vi "Base Ctrl Start Values.vi"(0 "Notifier Name In":string, 11 "Error In":errorcluster) -> (2 "Turret Filter":u32, 3 "Obj Index":u32, 4 "Notifier Name Out":string, 6 "Output Port":u32, 8 "Lamp Power":dbl, 10 "Lamp State":bool, 15 "Error Out":errorcluster)   [LabVIEW 2020]
uses:
  Device Library/Microscopes/Polymorphic Microscope Messenger/Get Turret Filter.vi
  Device Library/Microscopes/Polymorphic Microscope Messenger/Get Obj Index.vi
  Device Library/Microscopes/Polymorphic Microscope Messenger/Set Lamp Index.vi
  Device Library/Microscopes/Polymorphic Microscope Messenger/Get Output Port.vi
  Device Library/Microscopes/Polymorphic Microscope Messenger/Get Lamp Power.vi
  Device Library/Microscopes/Polymorphic Microscope Messenger/Get Lamp State.vi
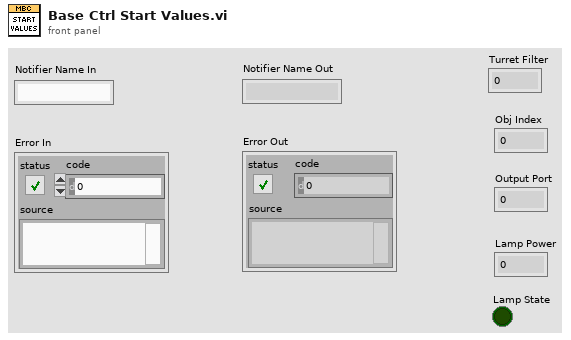
[diagram p1: front panel]
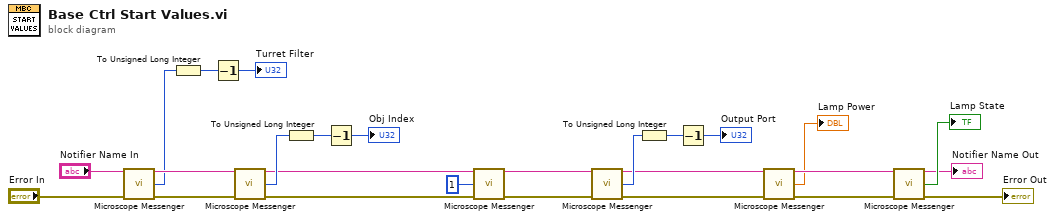
[diagram p0: block diagram]
diagram:
  n1 = call-poly "Microscope Messenger.vi"("Notifier Name In"="Notifier Name In", "Error In"="Error In") -> ("Notifier Name Out"=w19:string, "Turret Filter Index"=w17:u8, "Error Out"=w16:errorcluster)  [unwired: 11 in]
  n2 = To Unsigned Long Integer(number=w17) -> (unsigned 32bit integer=w18:u32)
  n3 = Decrement(x=w18) -> (x-1=→"Turret Filter":u32)
  n4 = call-poly "Microscope Messenger.vi"("Notifier Name In"=w19, "Error In"=w16) -> ("Notifier Name Out"=w25:string, "Objective Index"=w26:u8, "Error Out"=w15:errorcluster)  [unwired: 11 in]
  n5 = To Unsigned Long Integer(number=w26) -> (unsigned 32bit integer=w20:u32)
  n6 = Decrement(x=w20) -> (x-1=→"Obj Index":u32)
  n7 = call-poly "Microscope Messenger.vi"("Notifier Name In"=w25, "Lamp Index"=u8 1, "Error In"=w15) -> ("Notifier Name Out"=w23:string, "Error Out"=w14:errorcluster)  [unwired: 11 in]
  n8 = call-poly "Microscope Messenger.vi"("Notifier Name In"=w23, "Error In"=w14) -> ("Notifier Name Out"=w7:string, "Output Port"=w22:u8, "Error Out"=w6:errorcluster)  [unwired: 11 in]
  n9 = To Unsigned Long Integer(number=w22) -> (unsigned 32bit integer=w21:u32)
  n10 = Decrement(x=w21) -> (x-1=→"Output Port":u32)
  n11 = call-poly "Microscope Messenger.vi"("Notifier Name In"=w7, "Error In"=w6) -> ("Notifier Name Out"=w12:string, "Lamp Power (%)"=→"Lamp Power":dbl, "Error Out"=w13:errorcluster)  [unwired: 11 in]
  n12 = call-poly "Microscope Messenger.vi"("Notifier Name In"=w12, "Error In"=w13) -> ("Notifier Name Out"=→"Notifier Name Out":string, "Lamp State"=→"Lamp State":bool, "Error Out"=→"Error Out":errorcluster)  [unwired: 11 in]
